vi "Launch Editor.vi"() -> (0 "error out":errorcluster)   [LabVIEW 2020, in "Conditum-Tools.lvlib" / "Entity Editor.lvclass"]
uses:
  Entity Editor.lvclass
  Editor UI.vi
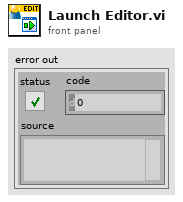
[diagram p1: front panel]
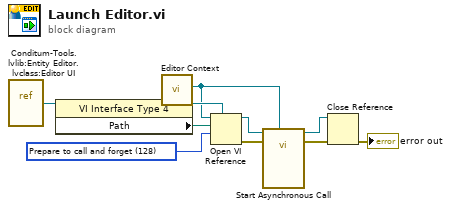
[diagram p0: block diagram]
diagram:
  w5 = 128 items=["Record modifications"=1, "Open templates for editing"=2, "Prompt user to save"=4, "Prepare for reentrant run"=8, "Prompt to find missing subVIs"=16, "Hide loading dialog box"=32, "Enable simultaneous calls"=64, "Prepare to call and forget"=128, "Simultaneous call and forget"=192, "Prepare to call and collect"=256, "Simultaneous call and collect"=320]
  n1 = vi-ref "Conditum-Tools.lvlib:Entity Editor.lvclass:Editor UI.vi"() -> (w3:refnum<vi>)
  n2 = property class="VI Interface Type 4"(reference=w3) -> (reference out=w6:refnum<vi>, "Path"=w4:path)  [unwired: 1 in, 1 out]
  n3 = call "Editor Context.vi"() -> ("Editor Context"=w1:refnum<vi>)  [unwired: 11 in]
  n4 = Open VI Reference(type specifier VI Refnum (for type only)=w6, application reference (local)=w1, vi path=w4, options=w5) -> (vi reference=w8:refnum<vi>, error out=w7:errorcluster)  [unwired: 2 in]
  n5 = call-by-ref "Start Asynchronous Call"(reference=w8, error in=w7, "Editor Context"=w1) -> (reference out=w10:refnum<vi>, error out=w9:errorcluster)  [unwired: 9 in, 2 out]
  n6 = Close Reference(reference=w10, error in (no error)=w9) -> (error out=→"error out":errorcluster)
